vi "Register for Waveform Data Events (DBL).vi"(8 "error in (no error)":errorcluster, 10 "WaveformStreamSpecifications":T3[](array[typedef]), 11 "WaveformStreaming in":T4) -> (0 "error out":errorcluster, 3 "WaveformStreaming out":T4, 4 "waveform data event registration (DBL)":refnum<event-registration>, 5 "registered waveform data event (DBL)":T1)   [LabVIEW 2020, in "NI_VS Waveform Streaming Interface.lvlib"]
doc: "Registers to receive waveform data from the specified <B>WaveformStreamSpecifications</B>. You can use this VI prior to starting waveform streams to generate an event registration refnum that allows an Event structure to stream data from waveforms. You must manually select the instance to use."
uses:
  <vilib>/NI VeriStand/Execution/WaveformStreaming/NI_VS Waveform Streaming Interface.lvlib
  <vilib>/NI VeriStand/Execution/WaveformStreaming/WaveformStreamingAPI.ctl
  NationalInstruments.VeriStand.ClientAPI
  <vilib>/NI VeriStand/Execution/WaveformStreaming/WaveformStreamSpecification.ctl
  <vilib>/NI VeriStand/Execution/WaveformStreaming/Registered Waveform Streams Data Event Refnum (DBL).ctl
  <vilib>/NI VeriStand/Execution/WaveformStreaming/Waveform Data Watcher Event Data (DBL).ctl
  <vilib>/NI VeriStand/Execution/WaveformStreaming/WaveformDataWatcherDBL.ctl
  <vilib>/NI VeriStand/Execution/WaveformStreaming/WaveformDataEventHandler Event Callback (DBL).vi
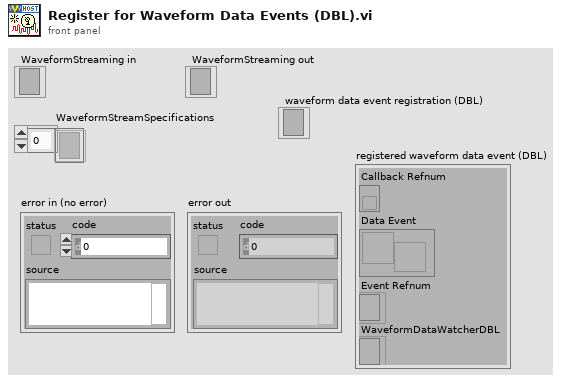
[diagram p1: front panel]
types:
  T1 = typedef "NI_VS Waveform Streaming Interface.lvlib/Registered Waveform Streams Data Event Refnum (DBL).ctl" = cluster{"Callback Refnum":refnum<k27>, "Data Event":refnum<user-event>, "Event Refnum":refnum<event-registration>, "WaveformDataWatcherDBL":T2}
  T2 = typedef "NI_VS Waveform Streaming Interface.lvlib/WaveformDataWatcherDBL.ctl" = refnum<k24>
  T3 = typedef "NI_VS Waveform Streaming Interface.lvlib/WaveformStreamSpecification.ctl" = refnum<k24>
  T4 = typedef "NI_VS Waveform Streaming Interface.lvlib/WaveformStreamingAPI.ctl" = refnum<k24>
  T5 = typedef "NI_VS Waveform Streaming Interface.lvlib/Waveform Data Watcher Event Data (DBL).ctl" = cluster{"Data":dbl[], "dt":dbl, "offset from start (samples)":u64, "t0 at start":timestamp, "WaveformStreamSpecification":T3}
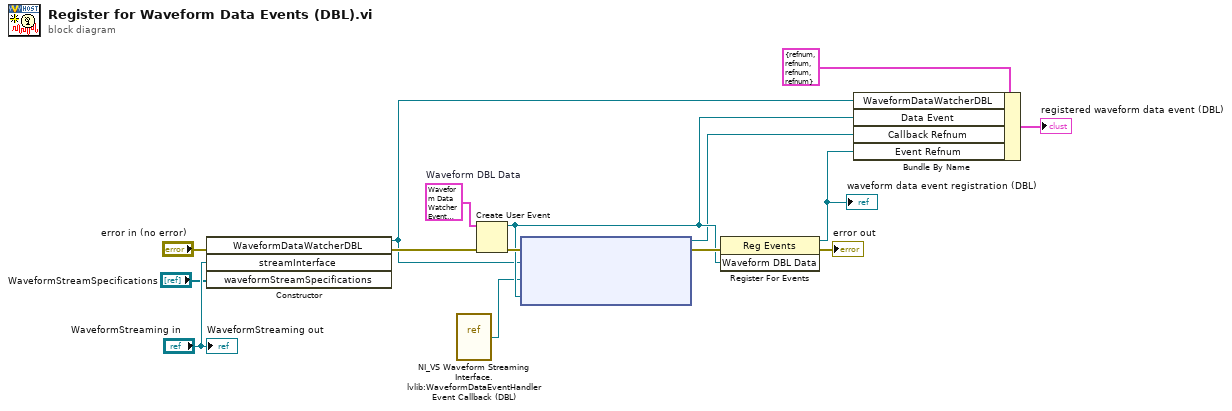
[diagram p0: block diagram]
diagram:
  w10 = T5 {"Data"=[], "dt"=0.0, "offset from start (samples)"=0, "t0 at start"=timestamp(0 s since 1904-01-01), "WaveformStreamSpecification"=refnum}  # Waveform DBL Data
  n1 = constructor class="WaveformDataWatcherDBL"(error in="error in (no error)", "streamInterface"="WaveformStreaming in", "waveformStreamSpecifications"="WaveformStreamSpecifications") -> (reference out=w2:refnum<k24>, error out=w13:errorcluster)  [unwired: 2 in, 3 out]
  n2 = vi-ref "NI_VS Waveform Streaming Interface.lvlib:WaveformDataEventHandler Event Callback (DBL).vi"() -> (w3:refnum<vi>)
  n3 = Create User Event(user event datatype=w10, error in=w13) -> (user event=w8:refnum<user-event>, error out=w12:errorcluster)
  n4 = node(w12, w2, w3, w8) -> (w4:refnum<k27>, w11:errorcluster)  [unwired: 1 in]
  n5 = register-events(error in=w11, w8) -> (reference out=w7:refnum<event-registration>, error out=→"error out":errorcluster)  [unwired: 1 in]
  "waveform data event registration (DBL)" <- w7
  n6 = Bundle By Name(cluster=T1 {"Callback Refnum"=refnum, "Data Event"=refnum, "Event Refnum"=refnum, "WaveformDataWatcherDBL"=refnum} ("Registered DBL Waveform Streams Data Event Refnum"), "WaveformDataWatcherDBL"=w2, "Data Event"=w8, "Callback Refnum"=w4, "Event Refnum"=w7) -> (→"registered waveform data event (DBL)":T1)
  "WaveformStreaming out" <- "WaveformStreaming in"
